vi "IMAGE ANALYSIS.vi"(7 "Enum":T1=enum."INIT", 8 "error in":errorcluster, 10 "IMAGE FILE PATH":string, 11 "File Path":path) -> (0 "error out":errorcluster, 3 "data out":string)   [LabVIEW 2025]
uses:
  POST ANALYSIS ENUM.ctl
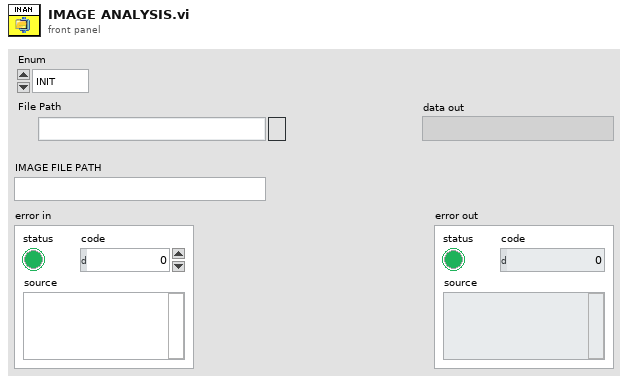
[diagram p1: front panel]
types:
  T1 = typedef "POST ANALYSIS ENUM.ctl" = enum16{"OPEN EXE", "INIT", "OPEN FILE", "FIT", "DRAW REC", "DRAW LINE", "PAN", "ZOOM IN", "ZOOM OUT", "SET ZOOM", "CLEAR ROI", "GET MEASUREMENTS", "RESIZE MODE", "STREAM START", "STREAM STOP", "SHOW UI", "MINIMIZE UI", "HIDE UI", "CKISE APP", "CLOSE CONNECTION", "SAVE IMAGE", "SET ROI COLOR", "READ", "TCP CHECK", "CLOSE"}
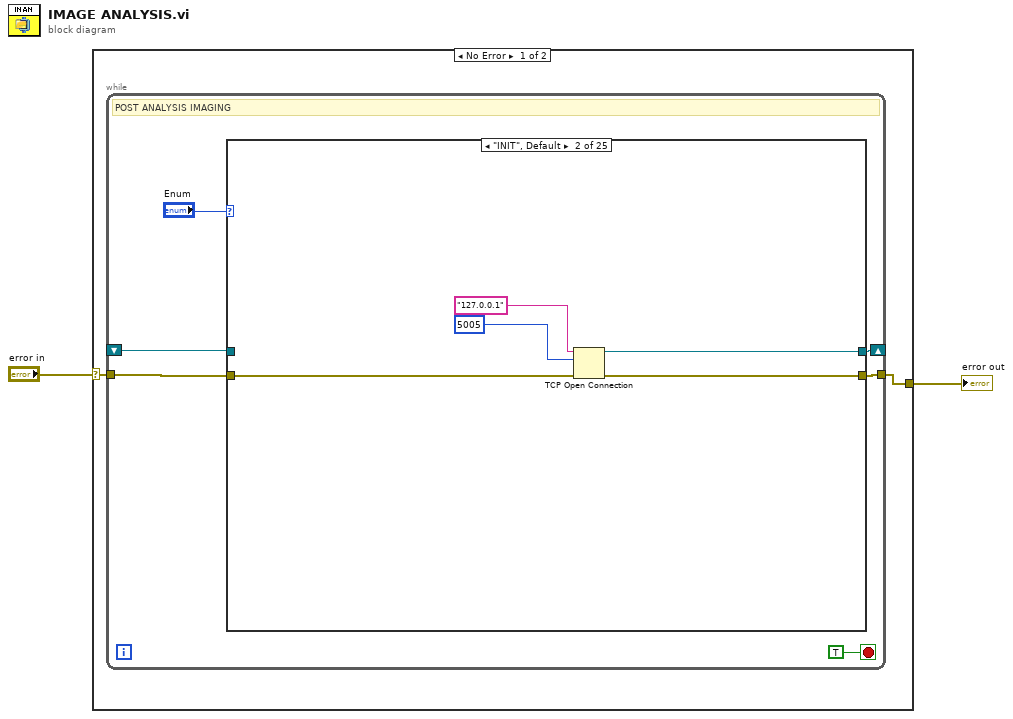
[diagram p0: block diagram]
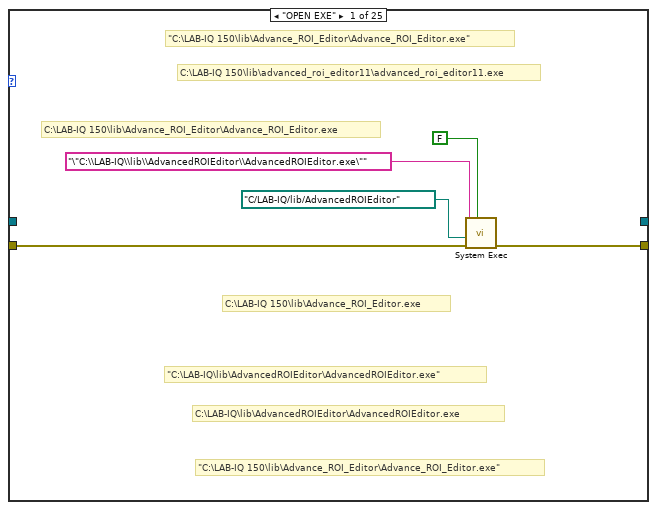
[diagram p2: hidden frame]
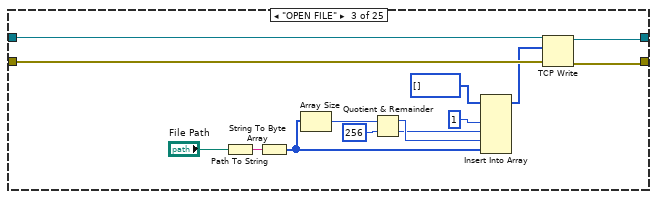
[diagram p3: hidden frame]
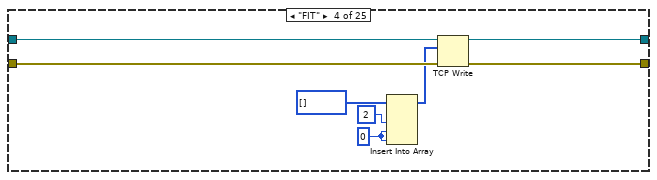
[diagram p4: hidden frame]
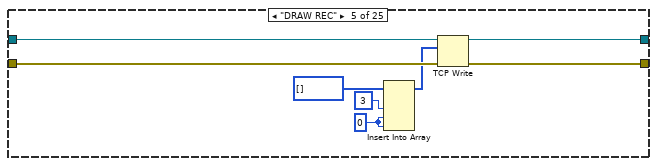
[diagram p5: hidden frame]
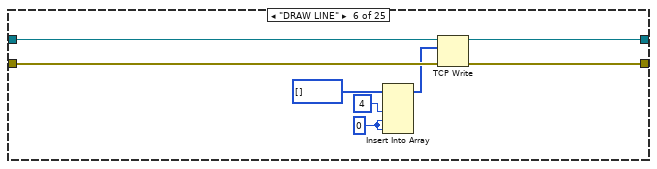
[diagram p6: hidden frame]
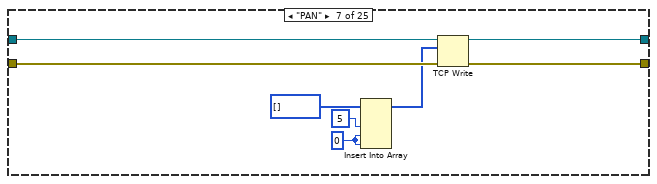
[diagram p7: hidden frame]
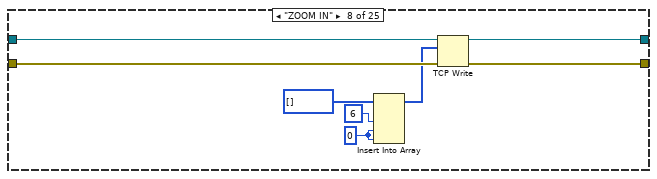
[diagram p8: hidden frame]
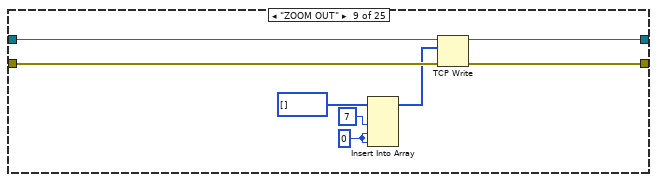
[diagram p9: hidden frame]
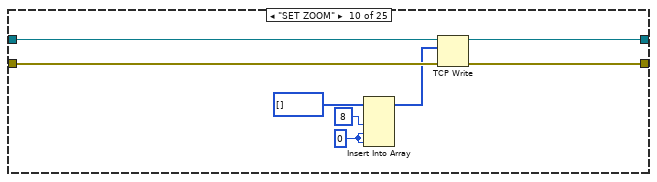
[diagram p10: hidden frame]
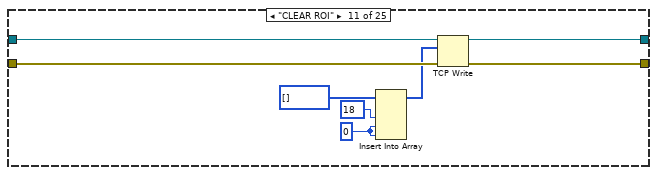
[diagram p11: hidden frame]
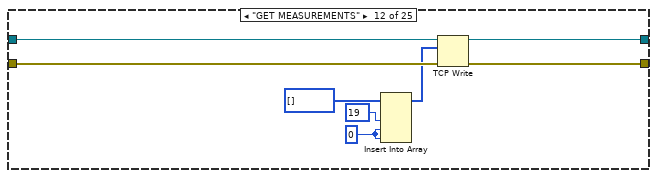
[diagram p12: hidden frame]
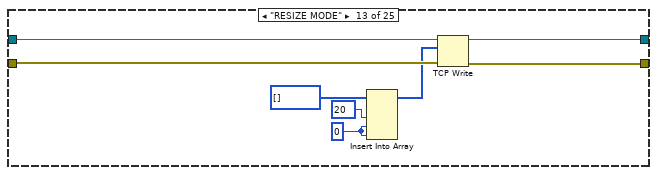
[diagram p13: hidden frame]
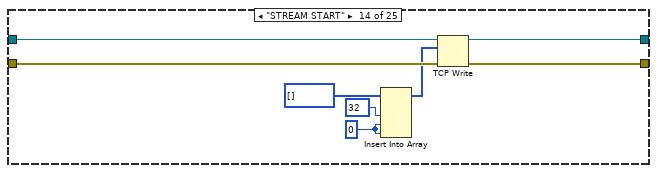
[diagram p14: hidden frame]
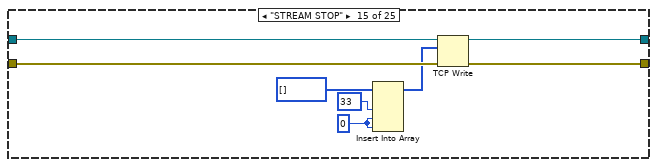
[diagram p15: hidden frame]
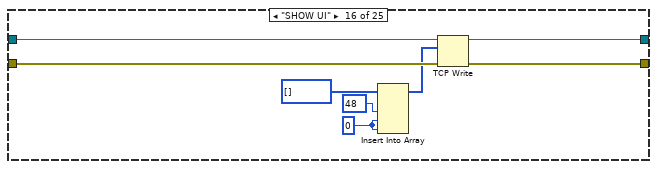
[diagram p16: hidden frame]
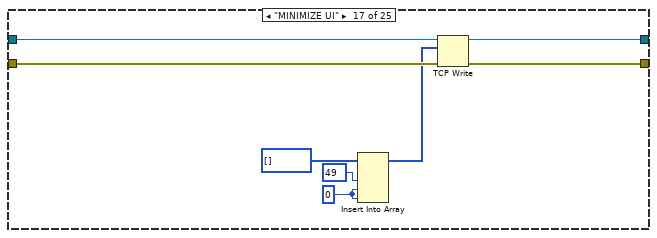
[diagram p17: hidden frame]
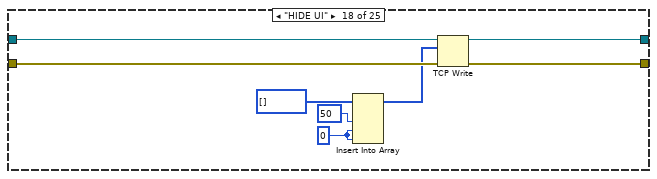
[diagram p18: hidden frame]
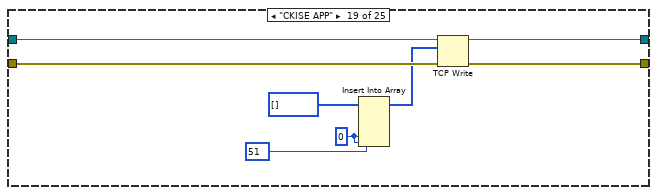
[diagram p19: hidden frame]
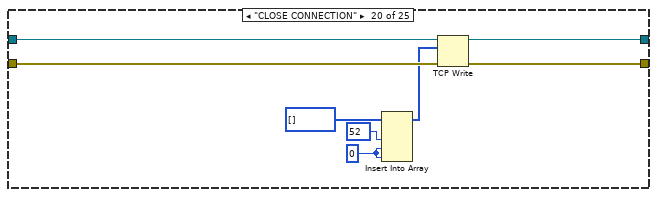
[diagram p20: hidden frame]
diagram:
  n1 = case shown="No Error" "error in" {
    selector: "error in" -> [w4 w212]
    tunnel: [w3 w211] -> w1
    frame No Error {
      n2 = while {
        tunnel: w4 -> [w8]
        tunnel: [w7] -> w3
        shift-right: [w6] -> _
        shift-left: _ -> [w5]
        stop <- TRUE stop-if-true
        # "POST ANALYSIS IMAGING"
        n3 = case shown="\"INIT\", Default" "Enum" {
          tunnel: w8 -> [w12 w18 w25 w39 w47 w55 w63 w71 w79 w87 w95 w103 w111 w119 w127 w135 w143 w151 w159 w167 w182 w188 w196 w207 w210]
          tunnel: [w11 w17 w24 w40 w48 w56 w64 w72 w80 w88 w96 w104 w112 w120 w128 w136 w144 w152 w160 w168 w183 w189 w197 w202 w209] -> w7
          tunnel: [_ w16 w22 w35 w43 w51 w59 w67 w75 w83 w91 w99 w107 w115 w123 w131 w139 w147 w155 w163 w180 w184 w192 w204 _] -> w6
          tunnel: w5 -> [_ _ w21 w36 w44 w52 w60 w68 w76 w84 w92 w100 w108 w116 w124 w132 w140 w148 w156 w164 w181 w185 w193 w206 w208]
          frame "OPEN EXE" {
            # "\"C:\\LAB-IQ 150\\lib\\Advance_ROI_Editor\\Advance_ROI_Editor.exe\""
            # "\"C:\\LAB-IQ\\lib\\AdvancedROIEditor\\AdvancedROIEditor.exe\""
            # "C:\\LAB-IQ\\lib\\AdvancedROIEditor\\AdvancedROIEditor.exe"
            # "C:\\LAB-IQ 150\\lib\\Advance_ROI_Editor\\Advance_ROI_Editor.exe"
            # "\"C:\\LAB-IQ 150\\lib\\Advance_ROI_Editor\\Advance_ROI_Editor.exe\""
            # "C:\\LAB-IQ 150\\lib\\advanced_roi_editor11\\advanced_roi_editor11.exe"
            # "C:\\LAB-IQ 150\\lib\\Advance_ROI_Editor.exe"
            n4 = call <vilib>:"System Exec.vi"("wait until completion? (T)"=FALSE, "error in (no error)"=w12, "working directory"=path "C:/LAB-IQ/lib/AdvancedROIEditor", "command line"="\"C:\\LAB-IQ\\lib\\AdvancedROIEditor\\AdvancedROIEditor.exe\"") -> ("error out"=w11:errorcluster)  [unwired: 4 in, 3 out]
          }
          frame "INIT", Default {
            n5 = TCP Open Connection(address="127.0.0.1", remote port or service name=u16 5005, error in (no error)=w18) -> (connection ID=w16:refnum<k5>, error out=w17:errorcluster)  [unwired: 2 in]
          }
          frame "OPEN FILE" {
            n6 = Path To String(path="File Path") -> (string=w27:string)
            n7 = String To Byte Array(string=w27) -> (unsigned byte array=w30:u8[])
            n8 = Array Size(array=w30) -> (size(s)=w32:i32)
            n9 = Quotient & Remainder(x=w32, y=256) -> (x-y*floor(x/y)=w29:i32, floor(x/y)=w28:i32)
            n10 = Insert Into Array(array=u8[] [] ("unsigned byte array"), new element #1=1, new element #2=w28, new element #3=w29, new element #4=w30) -> (w23:u8[])  [unwired: 1 in]
            n11 = TCP Write(connection ID=w21, data in=w23, error in (no error)=w25) -> (connection ID out=w22:refnum<k5>, error out=w24:errorcluster)  [unwired: 1 in, 1 out]
          }
          frame "FIT" {
            w41 = 0
            n12 = Insert Into Array(array=u8[] [] ("unsigned byte array"), new element #1=u8 2 ("new element/subarray"), new element #2=w41, new element #3=w41) -> (w37:u8[])  [unwired: 1 in]
            n13 = TCP Write(connection ID=w36, data in=w37, error in (no error)=w39) -> (connection ID out=w35:refnum<k5>, error out=w40:errorcluster)  [unwired: 1 in, 1 out]
          }
          frame "DRAW REC" {
            w49 = 0
            n14 = Insert Into Array(array=u8[] [] ("unsigned byte array"), new element #1=u8 3 ("new element/subarray"), new element #2=w49, new element #3=w49) -> (w45:u8[])  [unwired: 1 in]
            n15 = TCP Write(connection ID=w44, data in=w45, error in (no error)=w47) -> (connection ID out=w43:refnum<k5>, error out=w48:errorcluster)  [unwired: 1 in, 1 out]
          }
          frame "DRAW LINE" {
            w57 = 0
            n16 = Insert Into Array(array=u8[] [] ("unsigned byte array"), new element #1=u8 4 ("new element/subarray"), new element #2=w57, new element #3=w57) -> (w53:u8[])  [unwired: 1 in]
            n17 = TCP Write(connection ID=w52, data in=w53, error in (no error)=w55) -> (connection ID out=w51:refnum<k5>, error out=w56:errorcluster)  [unwired: 1 in, 1 out]
          }
          frame "PAN" {
            w65 = 0
            n18 = Insert Into Array(array=u8[] [] ("unsigned byte array"), new element #1=u8 5 ("new element/subarray"), new element #2=w65, new element #3=w65) -> (w61:u8[])  [unwired: 1 in]
            n19 = TCP Write(connection ID=w60, data in=w61, error in (no error)=w63) -> (connection ID out=w59:refnum<k5>, error out=w64:errorcluster)  [unwired: 1 in, 1 out]
          }
          frame "ZOOM IN" {
            w73 = 0
            n20 = Insert Into Array(array=u8[] [] ("unsigned byte array"), new element #1=u8 6 ("new element/subarray"), new element #2=w73, new element #3=w73) -> (w69:u8[])  [unwired: 1 in]
            n21 = TCP Write(connection ID=w68, data in=w69, error in (no error)=w71) -> (connection ID out=w67:refnum<k5>, error out=w72:errorcluster)  [unwired: 1 in, 1 out]
          }
          frame "ZOOM OUT" {
            w81 = 0
            n22 = Insert Into Array(array=u8[] [] ("unsigned byte array"), new element #1=u8 7 ("new element/subarray"), new element #2=w81, new element #3=w81) -> (w77:u8[])  [unwired: 1 in]
            n23 = TCP Write(connection ID=w76, data in=w77, error in (no error)=w79) -> (connection ID out=w75:refnum<k5>, error out=w80:errorcluster)  [unwired: 1 in, 1 out]
          }
          frame "SET ZOOM" {
            w89 = 0
            n24 = Insert Into Array(array=u8[] [] ("unsigned byte array"), new element #1=u8 8 ("new element/subarray"), new element #2=w89, new element #3=w89) -> (w85:u8[])  [unwired: 1 in]
            n25 = TCP Write(connection ID=w84, data in=w85, error in (no error)=w87) -> (connection ID out=w83:refnum<k5>, error out=w88:errorcluster)  [unwired: 1 in, 1 out]
          }
          frame "CLEAR ROI" {
            w97 = 0
            n26 = Insert Into Array(array=u8[] [] ("unsigned byte array"), new element #1=u8 18 ("new element/subarray"), new element #2=w97, new element #3=w97) -> (w93:u8[])  [unwired: 1 in]
            n27 = TCP Write(connection ID=w92, data in=w93, error in (no error)=w95) -> (connection ID out=w91:refnum<k5>, error out=w96:errorcluster)  [unwired: 1 in, 1 out]
          }
          frame "GET MEASUREMENTS" {
            w105 = 0
            n28 = Insert Into Array(array=u8[] [] ("unsigned byte array"), new element #1=u8 19 ("new element/subarray"), new element #2=w105, new element #3=w105) -> (w101:u8[])  [unwired: 1 in]
            n29 = TCP Write(connection ID=w100, data in=w101, error in (no error)=w103) -> (connection ID out=w99:refnum<k5>, error out=w104:errorcluster)  [unwired: 1 in, 1 out]
          }
          frame "RESIZE MODE" {
            w113 = 0
            n30 = Insert Into Array(array=u8[] [] ("unsigned byte array"), new element #1=u8 20 ("new element/subarray"), new element #2=w113, new element #3=w113) -> (w109:u8[])  [unwired: 1 in]
            n31 = TCP Write(connection ID=w108, data in=w109, error in (no error)=w111) -> (connection ID out=w107:refnum<k5>, error out=w112:errorcluster)  [unwired: 1 in, 1 out]
          }
          frame "STREAM START" {
            w121 = 0
            n32 = Insert Into Array(array=u8[] [] ("unsigned byte array"), new element #1=u8 32 ("new element/subarray"), new element #2=w121, new element #3=w121) -> (w117:u8[])  [unwired: 1 in]
            n33 = TCP Write(connection ID=w116, data in=w117, error in (no error)=w119) -> (connection ID out=w115:refnum<k5>, error out=w120:errorcluster)  [unwired: 1 in, 1 out]
          }
          frame "STREAM STOP" {
            w129 = 0
            n34 = Insert Into Array(array=u8[] [] ("unsigned byte array"), new element #1=u8 33 ("new element/subarray"), new element #2=w129, new element #3=w129) -> (w125:u8[])  [unwired: 1 in]
            n35 = TCP Write(connection ID=w124, data in=w125, error in (no error)=w127) -> (connection ID out=w123:refnum<k5>, error out=w128:errorcluster)  [unwired: 1 in, 1 out]
          }
          frame "SHOW UI" {
            w137 = 0
            n36 = Insert Into Array(array=u8[] [] ("unsigned byte array"), new element #1=u8 48 ("new element/subarray"), new element #2=w137, new element #3=w137) -> (w133:u8[])  [unwired: 1 in]
            n37 = TCP Write(connection ID=w132, data in=w133, error in (no error)=w135) -> (connection ID out=w131:refnum<k5>, error out=w136:errorcluster)  [unwired: 1 in, 1 out]
          }
          frame "MINIMIZE UI" {
            w145 = 0
            n38 = Insert Into Array(array=u8[] [] ("unsigned byte array"), new element #1=u8 49 ("new element/subarray"), new element #2=w145, new element #3=w145) -> (w141:u8[])  [unwired: 1 in]
            n39 = TCP Write(connection ID=w140, data in=w141, error in (no error)=w143) -> (connection ID out=w139:refnum<k5>, error out=w144:errorcluster)  [unwired: 1 in, 1 out]
          }
          frame "HIDE UI" {
            w153 = 0
            n40 = Insert Into Array(array=u8[] [] ("unsigned byte array"), new element #1=u8 50 ("new element/subarray"), new element #2=w153, new element #3=w153) -> (w149:u8[])  [unwired: 1 in]
            n41 = TCP Write(connection ID=w148, data in=w149, error in (no error)=w151) -> (connection ID out=w147:refnum<k5>, error out=w152:errorcluster)  [unwired: 1 in, 1 out]
          }
          frame "CKISE APP" {
            w161 = 0
            n42 = Insert Into Array(array=u8[] [] ("unsigned byte array"), new element #1=u8 51 ("new element/subarray"), new element #2=w161, new element #3=w161) -> (w157:u8[])  [unwired: 1 in]
            n43 = TCP Write(connection ID=w156, data in=w157, error in (no error)=w159) -> (connection ID out=w155:refnum<k5>, error out=w160:errorcluster)  [unwired: 1 in, 1 out]
          }
          frame "CLOSE CONNECTION" {
            w169 = 0
            n44 = Insert Into Array(array=u8[] [] ("unsigned byte array"), new element #1=u8 52 ("new element/subarray"), new element #2=w169, new element #3=w169) -> (w165:u8[])  [unwired: 1 in]
            n45 = TCP Write(connection ID=w164, data in=w165, error in (no error)=w167) -> (connection ID out=w163:refnum<k5>, error out=w168:errorcluster)  [unwired: 1 in, 1 out]
          }
          frame "SAVE IMAGE" {
            n46 = String To Byte Array(string="IMAGE FILE PATH") -> (unsigned byte array=w178:u8[])
            n47 = Array Size(array=w178) -> (size(s)=w179:i32)
            n48 = Quotient & Remainder(x=w179, y=256) -> (x-y*floor(x/y)=w177:i32, floor(x/y)=w176:i32)
            n49 = Insert Into Array(array=u8[] [] ("unsigned byte array"), new element #1=u8 22 ("new element/subarray"), new element #2=w176, new element #3=w177, new element #4=w178) -> (w171:u8[])  [unwired: 1 in]
            n50 = TCP Write(connection ID=w181, data in=w171, error in (no error)=w182) -> (connection ID out=w180:refnum<k5>, error out=w183:errorcluster)  [unwired: 1 in, 1 out]
          }
          frame "SET ROI COLOR" {
            w190 = 0
            n51 = Insert Into Array(array=u8[] [] ("unsigned byte array"), new element #1=u8 21 ("new element/subarray"), new element #2=w190, new element #3=w190) -> (w186:u8[])  [unwired: 1 in]
            n52 = TCP Write(connection ID=w185, data in=w186, error in (no error)=w188) -> (connection ID out=w184:refnum<k5>, error out=w189:errorcluster)  [unwired: 1 in, 1 out]
          }
          frame "TCP CHECK" {
            w198 = 0
            n53 = Insert Into Array(array=u8[] [] ("unsigned byte array"), new element #1=u8 0 ("new element/subarray"), new element #2=w198, new element #3=w198) -> (w194:u8[])  [unwired: 1 in]
            n54 = TCP Write(connection ID=w193, data in=w194, error in (no error)=w196) -> (connection ID out=w192:refnum<k5>, error out=w197:errorcluster)  [unwired: 1 in, 1 out]
          }
          frame "READ" {
            n55 = TCP Read(connection ID=w206, bytes to read=1000, error in (no error)=w207, 9:3000 ("timeout ms (25000)")) -> (connection ID out=w204:refnum<k5>, data out=→"data out":string, error out=w205:errorcluster)  [unwired: 1 in]
            n56 = call <vilib>:"Clear Errors.vi"("error in (no error)"=w205) -> ("error out"=w202:errorcluster)  [unwired: 5 in, 1 out]
          }
          frame "CLOSE" {
            n57 = TCP Close Connection(connection ID=w208, error in (no error)=w210) -> (error out=w209:errorcluster)  [unwired: 1 in, 1 out]
          }
        }
      }
    }
    frame Error {
      n58 = call <vilib>:"Clear Errors.vi"("error in (no error)"=w212) -> ("error out"=w211:errorcluster)  [unwired: 5 in, 1 out]
    }
  }
  "error out" <- w1
